vi "Constants.vi"() -> ()   [LabVIEW 2013, in "OPC UA Client Shared.lvlib"]
doc: "Use this Global VI to access the GUIDs assigned to the page resources of the Custom Device."
uses:
  OPC UA Client Shared.lvlib
panel:
  in  "Tab Control":enum32{"GUIDS", "Constants", "Properties"}(tab)
  in  "Data Tag_Write.GUID":string="ddff34a8-6f1a-4889-ab9a-0bec442b9af9"
  in  "Data Folder.GUID":string="6579feb5-1219-4a78-b605-46d71edd99ff"
  in  "Data Tag_Read.GUID":string="d90b1919-b5dd-4572-8e65-61ab77e1880c"
  in  "Tags.GUID":string="8ca7cb8f-b8e0-4777-98b2-189d42350187"
  in  "Status.GUID":string="7edfa8db-1108-4455-b477-d5a5949050b3"
  in  "OPC UA Client.GUID":string="b427fdee-6f3d-4280-85b2-59e4741516b9"
  in  "Tags.Name":string="Tags"
  in  "Status.Name":string="Status"
  in  "Connect.IP":string="IP"
  in  "Connect.Port":string="Connect.Port"
  in  "Connect.User":string="User"
  in  "Connect.Password":string="Password"
  in  "Connect.MessageMode":string="MessageMode"
  in  "Connect.Security":string="Security"
  in  "Connect.ClientCert.Public":string="ClientPublicCert"
  in  "Connect.ServerCert":string="ServerCert"
  in  "Connect.ClientCert.Private":string="ClientPrivateCert"
  in  "Channel.DataType":string="DataType"
  in  "Channel.TagPath":string="TagPath"
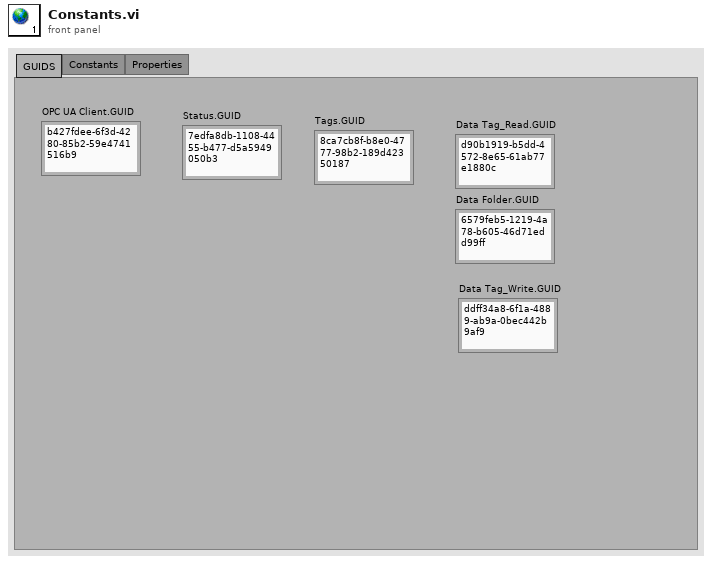
[diagram p1: front panel]
diagram:
